vi "Stop Page.vi"(9 "Operation":enum16{"Get", "Set"}(ring), 11 "user event":refnum<user-event>) -> (3 "user event (out)":refnum<user-event>)   [LabVIEW 2017, in "WebServiceImporter.lvlib" / "Main Panel.lvlib" / "Events.lvlib"]
uses:
  <vilib>/Platform/WebService/Main Panel/Events/Events.lvlib
  <vilib>/Platform/WebService/Main Panel/Events/Data Type/Page.ctl
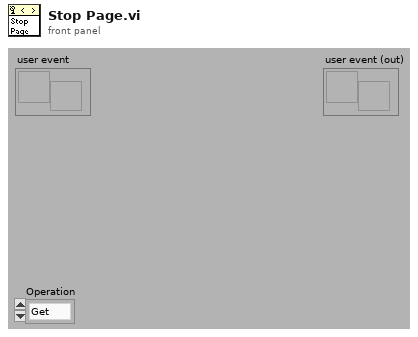
[diagram p1: front panel]
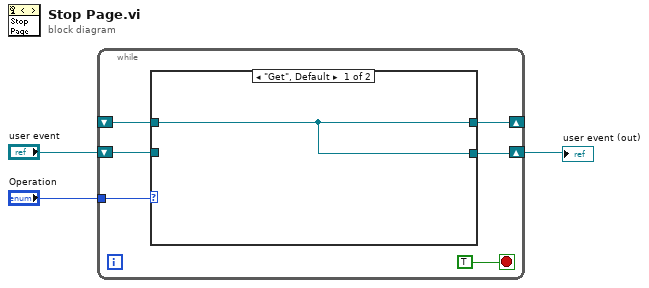
[diagram p0: block diagram]
diagram:
  n1 = while {
    tunnel: "Operation" -> [w9]
    shift-right: [w7] -> w1
    shift-left: "user event" -> [w8]
    shift-right: [w6] -> _
    shift-left: _ -> [w5]
    stop <- TRUE stop-if-true
    n2 = case shown="\"Get\", Default" w9 {
      tunnel: w8 -> [_ w11]
      tunnel: [w10 w11] -> w7
      tunnel: [w10 w11] -> w6
      tunnel: w5 -> [w10 _]
      frame "Get", Default {
      }
      frame "Set" {
      }
    }
  }
  "user event (out)" <- w1
